vi "Report Test Sequence.vi"() -> (2 "Sequence":refnum<class "Sequence Config.lvclass">)   [LabVIEW 2015, in "Sequencer Module tests.lvlib"]
uses:
  Sequencer Module tests.lvlib
  classes/Sequence/Config/Sequence Config.lvclass
  basic steps/Update Tag Step/Config/Update Tag Configuration/Update Tag Config.lvclass
  basic steps/Numeric Limit Compare/Config/Numeric Limit Compare Config.lvclass
  basic steps/Numeric Limit Compare/Config/Comparison Types.ctl
  <vilib>/NI/Tag Bus Module Framework/channel/channel classification.ctl
  <vilib>/NI/Tag Bus/tag/Data Type.ctl
  basic steps/Numeric Limit Compare/Config/Numeric Limit Compare Config.lvclass/Numeric Limit Compare Config.ctl
  basic steps/Numeric Limit Compare/Config/Write Comparison Type.vi
  basic steps/Numeric Limit Compare/Config/Write Lower Limit.vi
  basic steps/Numeric Limit Compare/Config/Write Negate Result.vi
  basic steps/Numeric Limit Compare/Config/Write Result Channel.vi
  basic steps/Numeric Limit Compare/Config/Write channel.vi
  basic steps/Numeric Limit Compare/Config/Write Upper Limit_Limit.vi
  <vilib>/NI/Tag Bus Module Framework/channel/TBM channel.lvclass
  <vilib>/NI/Tag Bus/tag/tag descriptor.lvclass
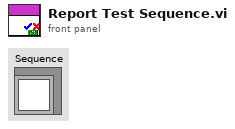
[diagram p1: front panel]
types:
  T1 = typedef "TBM channel.lvclass/channel classification.ctl" = enum16{"input data", "output data", "processing parameter", "processing result"}
  T2 = typedef "tag bus.lvlib/tag descriptor.lvclass/Data Type.ctl" = enum16{"Double", "Single", "I64", "I32", "I16", "I8", "U64", "U32", "U16", "U8", "Boolean", "String", "Array of Double", "Array of Single", "Array of I64", "Array of I32", "Array of I16", "Array of I8", "Array of U64", "Array of U32", "Array of U16", "Array of U8", "Array of Boolean", "Array of String"}
  T3 = typedef "Comparison Types.ctl" = enum16{"GELE (>=<=)", "GTLE(><=)", "GTLT(><)", "GELT(>=<)", "EQ(==)", "NE (!=)", "GT(>)", "LT(<)", "GE(>=)", "LE(<=)"}
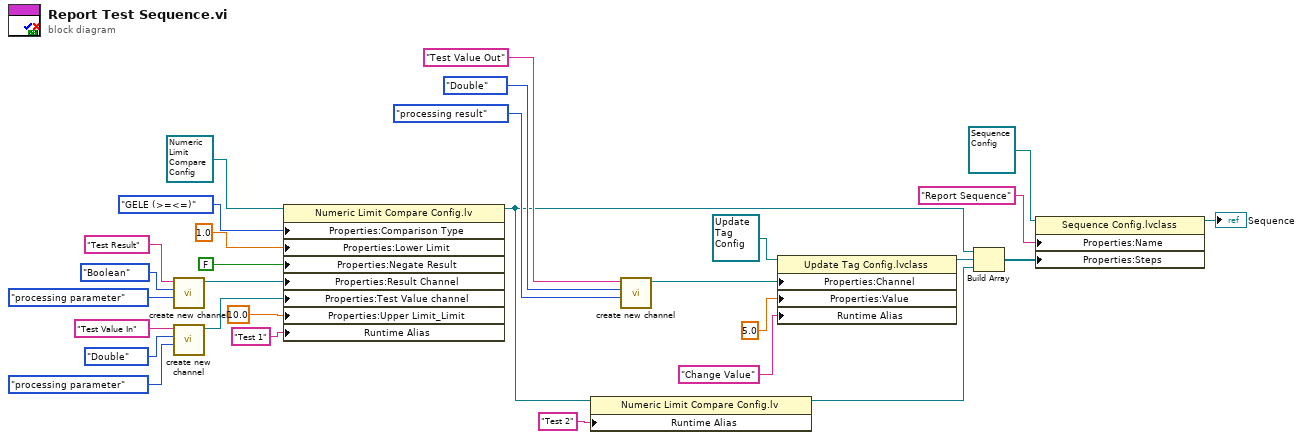
[diagram p0: block diagram]
diagram:
  n1 = call <vilib>:"create new channel.vi"("channel classification"=channel_classification."processing parameter", "data type"=Data_Type."Boolean", "channel name"="Test Result") -> ("channel"=w15:refnum<class "TBM channel.lvclass">)  [unwired: 8 in]
  n2 = call <vilib>:"create new channel.vi"("channel classification"=channel_classification."processing parameter", "data type"=Data_Type."Double", "channel name"="Test Value In") -> ("channel"=w6:refnum<class "TBM channel.lvclass">)  [unwired: 8 in]
  n3 = property class="Numeric Limit Compare Config.lv"(reference=refnum<class "Numeric Limit Compare Config.lvclass"> refnum ("Numeric Limit Compare Config.lvclass"), "Properties:Comparison Type"=Comparison_Types."GELE (>=<=)" ("Comparison Type"), "Properties:Lower Limit"=1.0 ("Lower Limit"), "Properties:Negate Result"=FALSE ("Negate Result"), "Properties:Result Channel"=w15, "Properties:Test Value channel"=w6, "Properties:Upper Limit_Limit"=10.0 ("Upper Limit_Limit"), "Runtime Alias"="Test 1") -> (reference out=w4:refnum<class "Numeric Limit Compare Config.lvclass">)  [unwired: 1 in, 1 out]
  n4 = property class="Numeric Limit Compare Config.lv"(reference=w4, "Runtime Alias"="Test 2") -> (reference out=w3:refnum<class "Numeric Limit Compare Config.lvclass">)  [unwired: 1 in, 1 out]
  n5 = call <vilib>:"create new channel.vi"("channel classification"=channel_classification."processing result", "data type"=Data_Type."Double", "channel name"="Test Value Out") -> ("channel"=w5:refnum<class "TBM channel.lvclass">)  [unwired: 8 in]
  n6 = property class="Update Tag Config.lvclass"(reference=refnum<class "Update Tag Config.lvclass"> refnum ("Update Tag Config.lvclass"), "Properties:Channel"=w5, "Properties:Value"=5.0 ("Upper Limit_Limit"), "Runtime Alias"="Change Value") -> (reference out=w11:refnum<class "Update Tag Config.lvclass">)  [unwired: 1 in, 1 out]
  n7 = Build Array(w4, w11, w3) -> (w12:refnum<class "Step Config.lvclass">[])
  n8 = property class="Sequence Config.lvclass"(reference=refnum<class "Sequence Config.lvclass"> refnum ("Sequence Config.lvclass"), "Properties:Name"="Report Sequence" ("Name"), "Properties:Steps"=w12) -> (reference out=→"Sequence":refnum<class "Sequence Config.lvclass">)  [unwired: 1 in, 1 out]
